vi "HindsPEM90_SetWavelength1.vi"(1 "Wavelength (nm)":dbl min=0.0 max=19999.9 step=0.1 format="%.1f", 5 "error in (no error)":errorcluster) -> (8 "Indicator":bool, 14 "VISA refnum out":refnum<visa-resource-name>, 19 "error out":errorcluster)   [LabVIEW 2016]
panel:
  in  "VISA refnum in":refnum<visa-resource-name>="COM1"
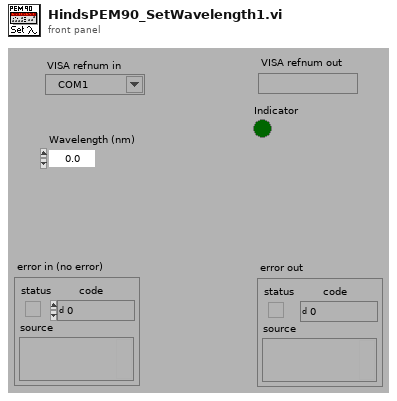
[diagram p1: front panel]
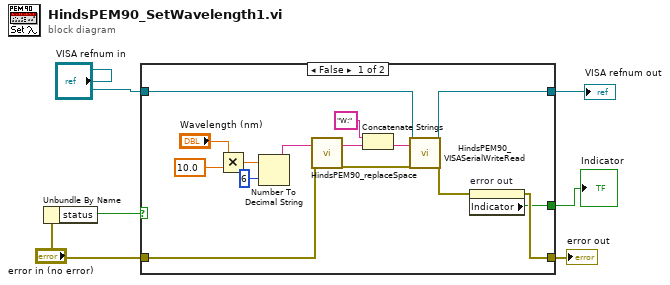
[diagram p0: block diagram]
diagram:
  n1 = Unbundle By Name("error in (no error)") -> ("status"=w6:bool)
  n2 = case shown="False" w6 {
    tunnel: "error in (no error)" -> [w18 w23]
    tunnel: [w8 w23] -> w4
    tunnel: "VISA refnum in" -> [w11 w22]
    tunnel: [w10 w22] -> w3
    tunnel: [w7 _] -> w2
    frame False {
      n3 = Multiply(x="Wavelength (nm)", y=10.0) -> (x*y=w16:dbl)
      n4 = Number To Decimal String(number=w16, width (-)=i16 6) -> (decimal integer string=w17:string)
      n5 = call "HindsPEM90_replaceSpace.vi"("Sting In"=w17, "error in (no error)"=w18) -> ("String Out"=w19:string, "error out"=w12:errorcluster)  [unwired: 16 in]
      n6 = Concatenate Strings("W:" ("Substring"), w19) -> (w21:string)
      n7 = call "HindsPEM90_VISASerialWriteRead.vi"("VISA refnum in"=w11, "write"=w21, "error in (no error)"=w12) -> ("VISA refnum out"=w10:refnum<visa-resource-name>, "error out"=w9:errorcluster)  [unwired: 14 in, 1 out]
      n8 = property on="error out" class="Clust (strict)"(error in=w9) -> (error out=w8:errorcluster, "Indicator"=w7:bool)  [unwired: 1 in, 1 out]
    }
    frame True {
    }
  }
  "error out" <- w4
  "VISA refnum out" <- w3
  "Indicator" <- w2
